vi "ReadStrains_v190627_A.vi"() -> ()   [LabVIEW 2017]
doc: "I. Description:\nThis example demonstrates how to make continuous, hardware-timed temperature measurement using a thermocouple.\n\nII. Instructions for Running:\n1. Specify the Physical Channel where you have connected the thermocouple.\n2. Enter the Minimum and Maximum temperature values in degrees C you expect to measure. A smaller range will allow a more accurate measurement.\n3. Enter the scan rate at which you want to run the acquisition.\n4. Specify the type of thermocouple you are using.\n5. Thermocouple measurements require cold-junction compensation (CJC) to correctly scale them. Specify the source of your cold-junction compensation.\n6. If your CJC source is \"Internal\", skip the rest of the steps.\n7. If your CJC source is \"Constant Value\", specify the value (usually room temperature) in degrees C.\n8. If your CJC source is \"Channel\", specify the CJC Channel name. \n9. Specify the appropriate Auto Zero Mode. See your device's hardware manual to find out if your device supports this attribute.\n\nIII. Block Diagram Steps:\n1. Create a Thermocouple (TC) temperature measurement channel.\n2. Get all the channels in the task.\n3. Convert channel(s) array to a comma-delimited channel string.\n4. This attribute is set to compensate for input offset errors. May not be supported by all devices*.\n5. Call the Timing VI to specify the hardware timing parameters. Use device's internal clock, continuous mode acquisition and the sample rate specified by the user.\n6. Call the Start VI to program and start the acquisition.\n7. Read N samples and plot it. By default, the Read VI reads all available samples, but you can specify how many samples to read at a time and the timeout value. Continue reading data until the stop button is pressed or an error occurs. \n8. Call the Clear Task VI to clear the Task.\n9. Use the popup dialog box to display an error if any.\n\n* If your device does not support Auto Zero Mode bypass Step 2, 3, and 4.\n\nIV. I/O Connections Overview:\nConnect your thermocouple to the terminals corresponding to the Physical Channel I/O Control value."
uses:
  <vilib>/Utility/error.llb/DialogType.ctl
  <vilib>/DAQmx/read.llb/DAQmx Read (Counter DBL 1Chan 1Samp).vi
  <vilib>/DAQmx/write.llb/DAQmx Write (Digital 1D Bool NChan 1Samp 1Line).vi
  <vilib>/DAQmx/read.llb/DAQmx Read (Analog 1D Wfm NChan NSamp).vi
  <vilib>/Analysis/baseanly.llb/Mean (DBL).vi
  <vilib>/DAQmx/create/channels.llb/DAQmx Create Channel (DO-Digital Output).vi
  <vilib>/Waveform/WDTOps.llb/WDT Index Channel DBL.vi
  <vilib>/DAQmx/create/channels.llb/DAQmx Create Channel (AI-Voltage-Basic).vi
  <vilib>/DAQmx/configure/timing.llb/DAQmx Timing (Sample Clock).vi
  <vilib>/DAQmx/create/channels.llb/DAQmx Create Channel (CI-Frequency).vi
  <vilib>/DAQmx/miscellaneous.llb/DAQmx Fill In Error Info.vi
  <vilib>/express/express arith-compare/Formula/XNode/ExpressFormulaBlockNode.xnode
  <vilib>/Analysis/NI_AALBase.lvlib
  <vilib>/ptbypt/NI_PtbyPt.lvlib
  <vilib>/Utility/miscctls.llb/LVRowAndColumnTypeDef.ctl
  <resource>/objmgr/daqmx.rc
panel:
  out "abs(x)":dbl
  in  "Min Frequency":dbl=0.1 format="%0.6f"
  in  "Max Frequency":dbl=50000.0 format="%0.6f"
  in  "Frequency Input Terminal":tag="/Dev1/PFI1"
  out "Freq (Hz)":dbl=5258.660356274239
  in  "Stop":bool
  in  "Counter":tag="Dev1/ctr0"
  in  "Color Box":u32(colorbox)=16448250
  out "Micro-strain":dbl[](array[numeric]) format="%.2g"
  out "Results":i32[](listbox)
  in  "num_chans":i32=4
  in  "Search Strings":string[](array[string])=["Verbose Name", "Units", "Sensitivity", "Offset"]
  out "TRQ_2SPD_OT (N·m)":dbl=-0.01305389404296875 format="%0.3f"
  out "Power_OT (W)":dbl=-4.779110606064606 format="%.2f"
  out "rpm_out/rpm_in":dbl=-8.382425226893735e-05 format="%.3g"
  out "switch_counts":dbl=4500000.0
  in  "switch_time (s)":dbl=900000.0
  out "AI Consumer Iterations":i32=46
  in  "LV_CMD_2SPD_OIL_SLND":bool[](array[boolean])=[FALSE]
  in  "lines":tag="Dev1/port1/line0"
  out "RPM_2SPD_OT_6602":dbl format="%0.1f"
  in  "path":path=path "D:/LabView Data"
  in  "DRVLN_PULLEY_RATIO":dbl=1.48 format="%.2f"
  out "P2 - P1":dbl=2.2560862731933593 format="%.3f"
  out "Recorded Blocks":dbl=46.0
  out "AI Producer Iterations":i32=45
  in  "Force Record":bool caption="Force Record Enable"
  out "RPM_DRVLN_6602":dbl format="%0.1f"
  out "data 2":waveform(dbl)[](array[waveform])=[{"t0"=timestamp(3650018127.9917235 s since 1904-01-01), "dt"=0.1, "Y"=[0.021594634133905076, 0.022275858634939055], "attributes"=variant("NI_ChannelName"=variant(string "Dev1/ai0"), "NI_UnitDescription"=variant(string "Volts"))}, {"t0"=timestamp(3650018127.9917235 s since 1904-01-01), "dt"=0.1, "Y"=[2.0002340930725198, 1.9998772609501023], "attributes"=variant("NI_ChannelName"=variant(string "Dev1/ai0"), "NI_UnitDescription"=variant(string "Volts"))}, {"t0"=timestamp(3650018127.9917235 s since 1904-01-01), "dt"=0.1, "Y"=[1.9878001157523826, 1.9871643057998443], "attributes"=variant("NI_ChannelName"=variant(string "Dev1/ai0"), "NI_UnitDescription"=variant(string "Volts"))}, {"t0"=timestamp(3650018127.9917235 s since 1904-01-01), "dt"=0.1, "Y"=[0.006912624203864532, 0.006889916720453561], "attributes"=variant("NI_ChannelName"=variant(string "Dev1/ai0"), "NI_UnitDescription"=variant(string "Volts"))}, {"t0"=timestamp(3650018127.9917235 s since 1904-01-01), "dt"=0.1, "Y"=[0.0, 0.0], "attributes"=variant("NI_ChannelName"=variant(string "Dev1/ai0"), "NI_UnitDescription"=variant(string "Volts"))}]
  out "Power_IN (W)":dbl=0.0005711775684961294 format="%.2g"
  out "TRQ_2SPD_DRVLN_OT (N·m)":dbl=-0.018612060546874976 format="%0.3f"
  out "Waveform Chart":waveform(dbl)[](graph)=[{"t0"=timestamp(3663084502.027375 s since 1904-01-01), "dt"=0.1, "Y"=[-0.17066702696318498, -0.13693019437081472], "attributes"=variant("NI_ChannelName"=variant(string "HS_2210_STRAIN_A_POUNDS"), "NI_UnitDescription"=variant(string "lbf"))}, {"t0"=timestamp(3663084502.027375 s since 1904-01-01), "dt"=0.1, "Y"=[-50.01120067249004, -50.01071408355846], "attributes"=variant("NI_ChannelName"=variant(string "T1_OIL_OT"), "NI_UnitDescription"=variant(string "°C"))}, {"t0"=timestamp(3663084502.027375 s since 1904-01-01), "dt"=0.1, "Y"=[-0.013838771793185324, -0.013803088604682188], "attributes"=variant("NI_ChannelName"=variant(string "HS_2210_STRAIN_B_VOLTS"), "NI_UnitDescription"=variant(string "V"))}, {"t0"=timestamp(3663084502.027375 s since 1904-01-01), "dt"=0.1, "Y"=[10.033860995992347, 10.033912900500356], "attributes"=variant("NI_ChannelName"=variant(string "HS_2210_EXC_B_VOLTS"), "NI_UnitDescription"=variant(string "V"))}, {"t0"=timestamp(3663084502.027375 s since 1904-01-01), "dt"=0.1, "Y"=[1.48, 1.48], "attributes"=variant("NI_ChannelName"=variant(string "RPM_RATIO"), "NI_UnitDescription"=variant(string "ratio"))}, {"t0"=timestamp(3663084502.027375 s since 1904-01-01), "dt"=0.1, "Y"=[99.0, 99.0], "attributes"=variant("NI_ChannelName"=variant(string "DataTag"), "NI_UnitDescription"=variant(string "none"))}, {"t0"=timestamp(3663084502.027375 s since 1904-01-01), "dt"=0.1, "Y"=[0.0, 0.0], "attributes"=variant("NI_ChannelName"=variant(string "LV_CMD_2SPD_OIL_SLND"), "NI_UnitDescription"=variant(string "boolean"))}]
  in  "Run Letter":string="a"
  out "Recording":bool
  in  "Num_Blocks":dbl=100.0
  in  "Data Tag":dbl=99.0 format="%.2p"
  in  "Maximum Value":dbl=10.0 format="%0.2f"
  in  "Minimum Value":dbl=-10.0 format="%0.2f"
  in  "Physical Channel":tag="Dev1/ai0:3" caption="PCI-6143_1 Channels"
  in  "Rate":dbl=1000.0 format="%0.2f"
  # "rev 150415_A  added \"Record Run X\" sub VI.\nrev 150423_A added power, efficiency, and manual inputs for speed .\nrev 150423_B added speed measurement via PCI-6602 card.\nrev 161117_A is set up for the alternator test reading shaft RPM from Dynapar encoder and torque from the Omega TQ513-1K paired with the Omega DP41-S.\nrev 170504_A migrated DAQ h/w from the SCXI chassis (now being used for TC2 porcupine testing) to PCI-6143.\nrev 170510_A takes data at 1000Hz, then averages groups of 100 samples for a logging rate of 10Hz per channel.  Added function that resets \"Data Tag\"\nto 99 after \"Num_Blocks\" has been recorded.\nrev 170810_A adds flowmeter for 2-speed supercharger drive bench test.  CJP\nrev 170821_A logs tags to same file for a given run letter.  Uses \"Record Continuous Tags...\" sub VI.\nrev 171129_A is for the Orthrus 2-speed drive.  Added new encoder period measurement for the 127 tooth geat \"RPM_2SPD_OT\". CJP\nrev 171130_A adds Digital Output (DO) for 2SPD drive control.  Will log this with the rest of the data.  Also corrected the number of teeth on the 2SPD Output side from 127 to 107!\nrev 171201_A restructuring for  \"real-time\" response to speed changes by moving the disklog to a separate loop (queue).\nrev 171201_B moves counters into main AI loop and adds a start trigger so DAQ won't start until rig is spinning.  Added F-V where old \"F1\" channel was for \"RPM_2SPD_OT\".   CJP\nrev 171201_C uses a CI-Frequency task for RPM instead of period.  Testing this for better transient response.  This appears to be even slower than the period measurement.\nrev 171201_D is built from rev 171201_A, but adding in the F-V channel.  This version queues both the AI channel and CI channels to a single Consumer.  Also adding a 30s switch to automate switching of the 2SPD solenoid.\nrev 171221_A was the first attempt at this and for some reason, while running that VI, the computer froze, unable to do ctrl+alt+del reboot.  After rebooting, the VI was no longer openable in LabView 2014 or LabView 2016.  Will try the same process over with v171226_A.\nrev 171226_A adds one more PCI_6143 card for 8 additional analog inputs.\nrev 171226_B created a backup with 171226_A.\nrev 180314_A added thermocouple for Sumanth.  This is for testing the 2-Speed Drive.\nrev Read \"ThermVolt_TestSpeed_180406_A.vi\" is for verifying the one remaining Micro-Epsilon speed sensor on the 2Spd Drive.\nrev \"Read Thermocouples and Voltages v180406_A.vi\" reintroduces the two counter/timer channels on the PCI-6602 card for the driveline encoder and \nMicro-Epsilon 2Spd Output.\nrev 180919_A built off of rev 180426_A for 2-Speed Drive testing.  CJP\nv181002_A adding new T22 at 2SPD input pulley AND keeping original T22 at output end of drivline.  CJP\nv181004_A corrected front panel displays for Power_IN and Power_OT.  CJP\nv181025_A adding ReadChnCfg.VI to read channel names, units, scaling, and offset from Labview Channel Map\nv190401_A restructuring \"Read Thermocouples and Voltages...\" to use only channels from NI-6229 out of test cell 2.  CJP\nv190516_A adds frequency measurement for driveline speed since F-V measurements not working.  CJP"
  # "For instructions, select Help>>Show Context Help"
  # "Now using 360 PPR encoder for input speed 171227.\nChanged to Input Gear Speed 180118.  CJP  127 Hz = 1 RPS, 127 Hz = 60 RPM\n5 kHz = 1 V => 5000/127 = 39.37 RPS = 2362.205 RPM\nv180314_A 5kHz = 1V = 5000/360 = 13.888 RPS = 833.33 RPM.\nBack to 360PPR encoder with pulley ratio of 1.48."
  # "HBM T21WN"
  # "Interface T22"
  # "Timing Parameters"
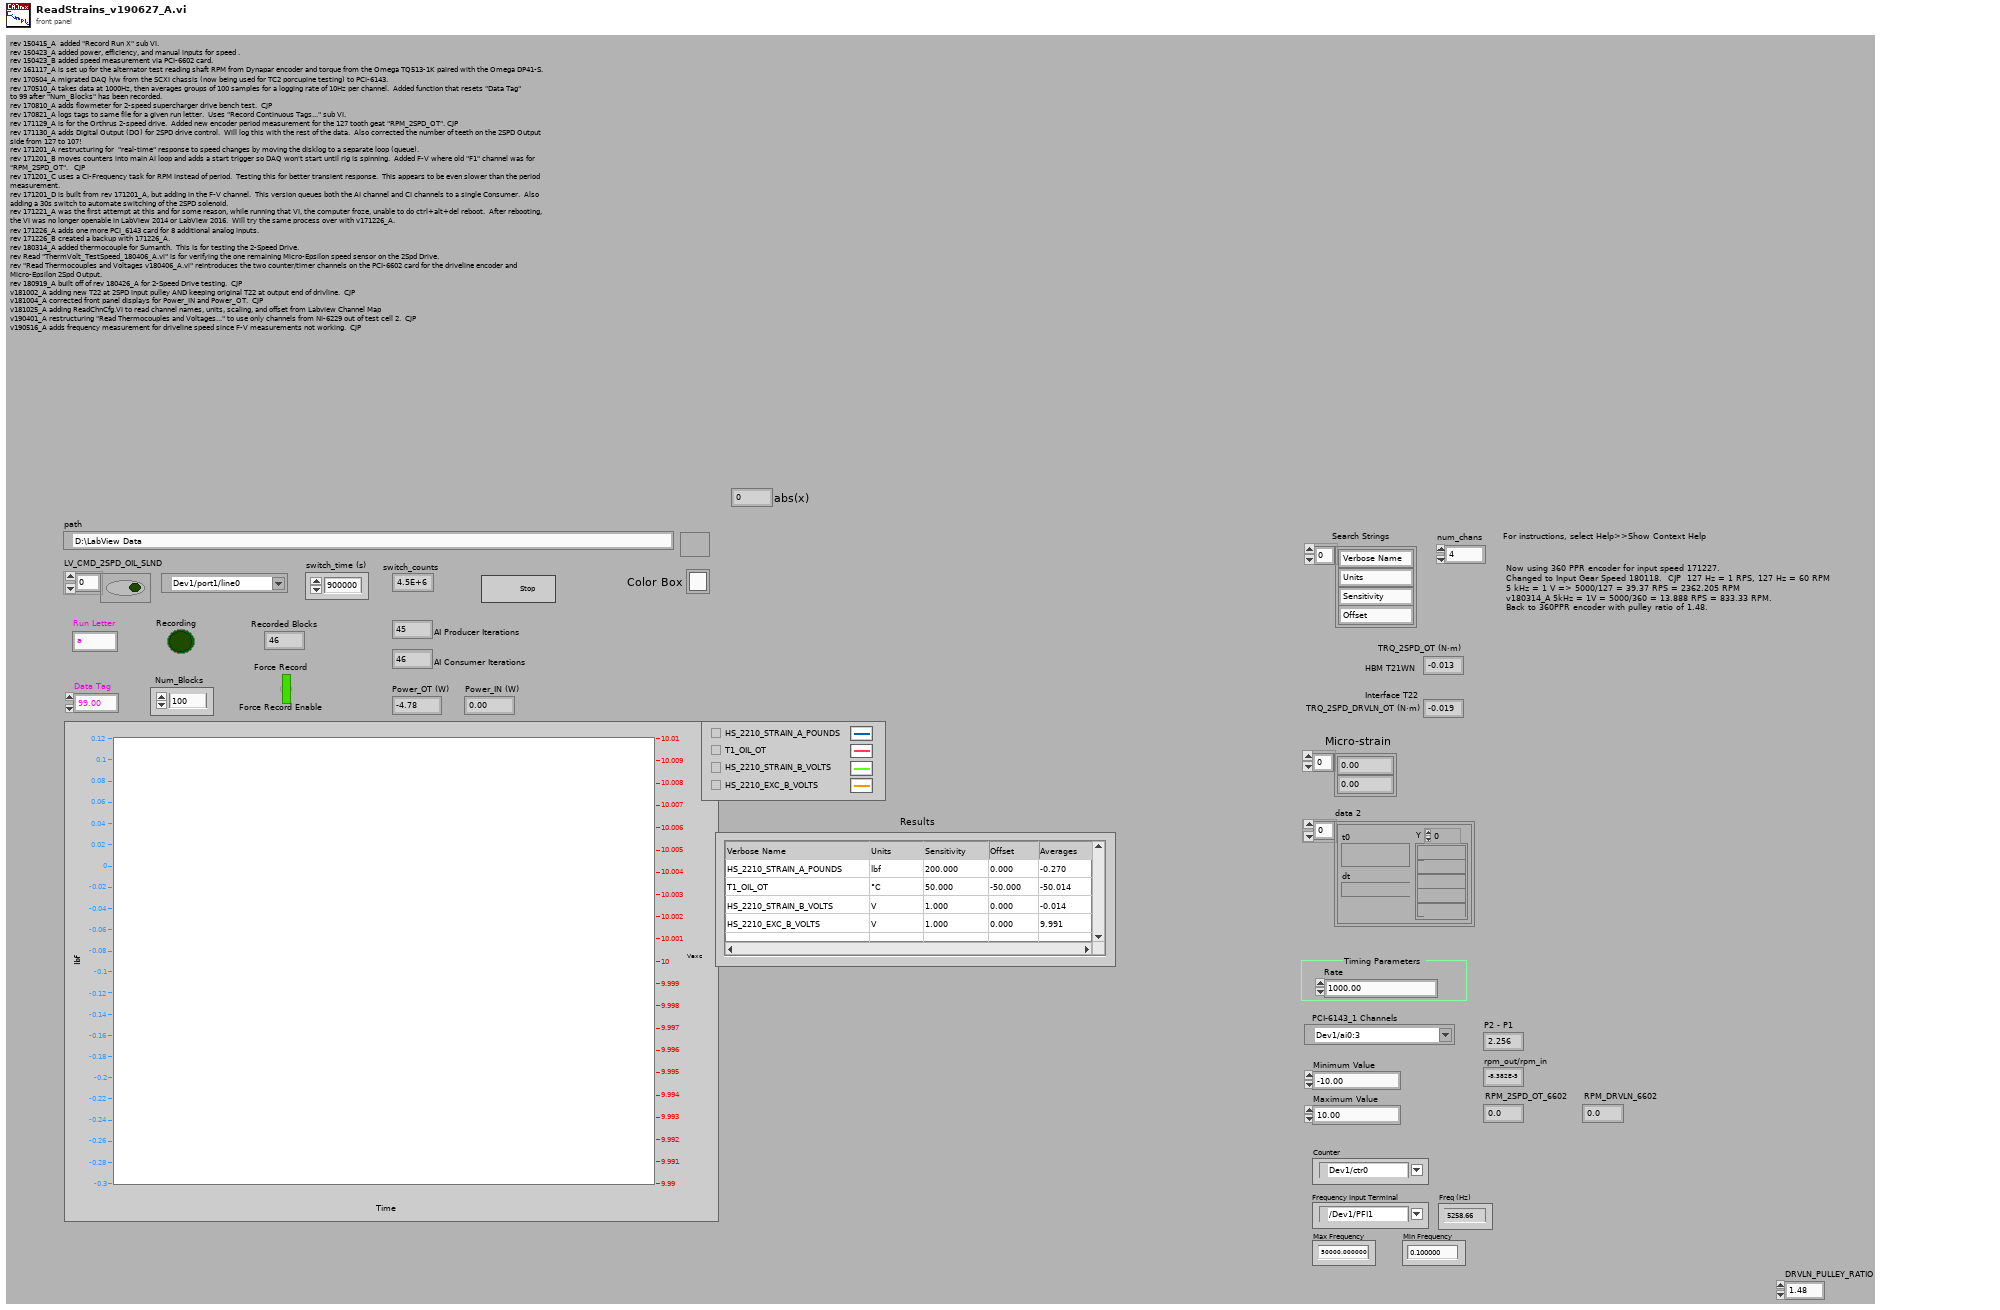
[diagram p1: front panel]
types:
  T1 = typedef "DialogType.ctl" = u16
  T2 = typedef "LVRowAndColumnTypeDef.ctl" = cluster{"Row":i32, "Column":i32}
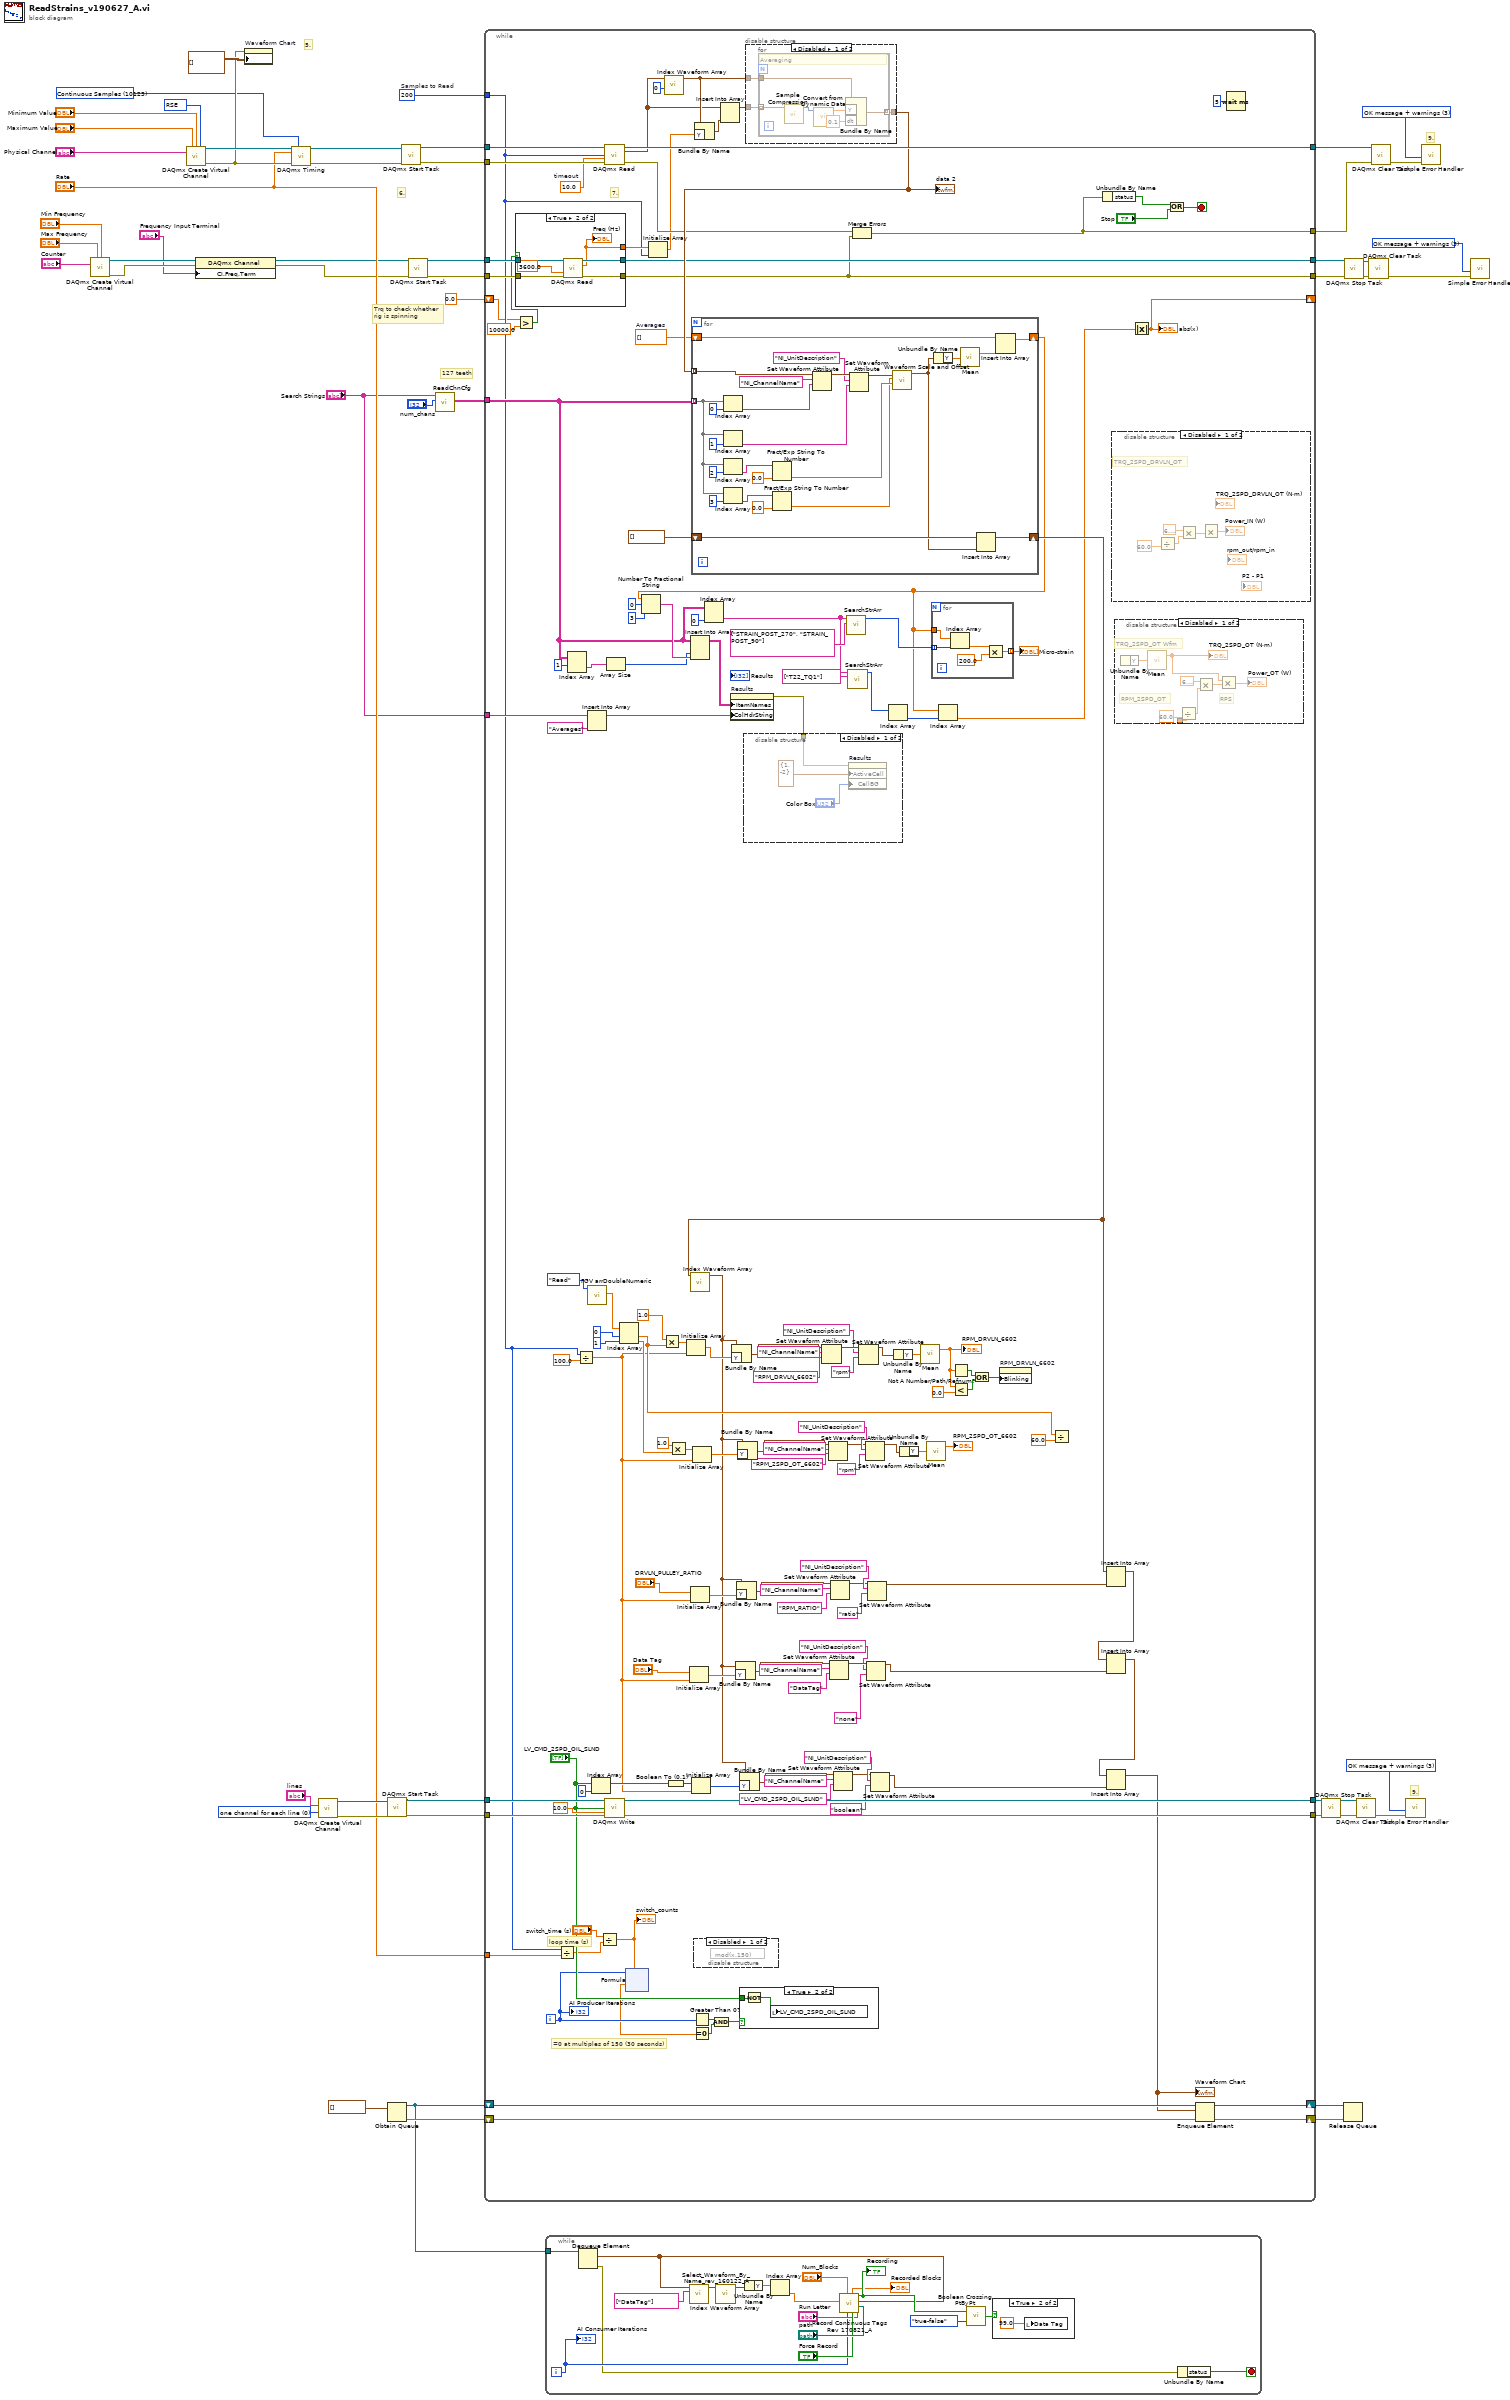
[diagram p0: block diagram]
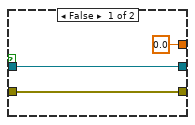
[diagram p4: hidden frame]
diagram:
  w11 = T1 3 items=["no dialog", "OK message", "continue or stop message", "OK message + warnings", "continue/stop + warnings"] ("type of dialog (OK msg:1)")
  w18 = 10083 items=["Default"=-1, "RSE"=10083, "NRSE"=10078, "Differential"=10106, "Pseudodifferential"=12529] ("input terminal configuration")
  w38 = T1 3 items=["no dialog", "OK message", "continue or stop message", "OK message + warnings", "continue/stop + warnings"] ("type of dialog (OK msg:1)")
  w44 = 0 items=["one channel for each line", "one channel for all lines"] ("line grouping")
  w50 = T1 3 items=["no dialog", "OK message", "continue or stop message", "OK message + warnings", "continue/stop + warnings"] ("type of dialog (OK msg:1)")
  w24 = 10123 items=["Finite Samples"=10178, "Continuous Samples"=10123] ("sample mode")
  # "Trq to check whether\nrig is spinning"
  # "127 teeth"
  # "Samples to Read"
  # "9."
  # "9."
  # "5."
  # "6."
  n1 = call-poly <vilib>:"DAQmx Create Virtual Channel.vi"("maximum value"="Max Frequency", "minimum value"="Min Frequency", "counter"="Counter") -> ("task out"=w10:refnum<k21>, "error out"=w9:errorcluster)  [unwired: 11 in]
  n2 = call-poly <vilib>:"DAQmx Create Virtual Channel.vi"("maximum value"="Maximum Value", "minimum value"="Minimum Value", "input terminal configuration"=w18, "physical channels"="Physical Channel") -> ("task out"=w48:refnum<k21>, "error out"=w46:errorcluster)  [unwired: 10 in]
  n3 = property class="DAQmx Channel"(reference=w10, error in=w9, "CI.Freq.Term"="Frequency Input Terminal") -> (reference out=w15:refnum<k21>, error out=w16:errorcluster)
  n4 = property on="Waveform Chart" class="WFChart (strict)"(error in=w46, "History Data"=waveform(dbl)[][] []) -> ()  [unwired: 1 in, 2 out]
  n5 = call-poly <vilib>:"DAQmx Timing.vi"("task/channels in"=w48, "sample mode"=w24, "rate"="Rate", "error in"=w46) -> ("task out"=w51:refnum<k21>, "error out"=w19:errorcluster)  [unwired: 10 in]
  n6 = call-poly <vilib>:"DAQmx Create Virtual Channel.vi"("lines"="lines", "line grouping"=w44) -> ("task out"=w43:refnum<k21>, "error out"=w42:errorcluster)  [unwired: 12 in]
  n7 = call <vilib>:"DAQmx Start Task.vi"("task/channels in"=w43, "error in"=w42) -> ("task out"=w41:refnum<k21>, "error out"=w40:errorcluster)  [unwired: 12 in]
  n8 = Obtain Queue(element data type=waveform(dbl)[] [] ("appended array")) -> (queue out=w28:refnum<queue>, error out=w31:errorcluster)  [unwired: 4 in, 1 out]
  n9 = call <vilib>:"DAQmx Start Task.vi"("task/channels in"=w51, "error in"=w19) -> ("task out"=w53:refnum<k21>, "error out"=w54:errorcluster)  [unwired: 12 in]
  n10 = call <vilib>:"DAQmx Start Task.vi"("task/channels in"=w15, "error in"=w16) -> ("task out"=w5:refnum<k21>, "error out"=w4:errorcluster)  [unwired: 12 in]
  n11 = call "ReadChnCfg.vi"("num_chans"="num_chans", "Search Strings"="Search Strings") -> ("Table Minus Headers"=w22:string[][])  [unwired: 8 in, 1 out]
  n12 = while {
    tunnel: w53 -> [w196]
    tunnel: w54 -> [w195]
    tunnel: [w194] -> w52
    tunnel: 200 ("number of samples per channel") -> [w71]
    tunnel: w41 -> [w142]
    tunnel: w40 -> [w141]
    tunnel: [w140] -> w35
    tunnel: [w139] -> w34
    shift-right: [w125] -> w30
    shift-left: w28 -> [w127]
    shift-right: [w124] -> w29
    shift-left: w31 -> [w126]
    tunnel: "Rate" -> [w118]
    tunnel: [w76] -> w20
    tunnel: w22 -> [w85]
    tunnel: "Search Strings" -> [w95]
    tunnel: w5 -> [w79]
    tunnel: w4 -> [w78]
    tunnel: [w75] -> w3
    tunnel: [w74] -> w2
    shift-right: [w59] -> _
    shift-left: 0.0 -> [w58]
    i -> [w115]
    stop <- w191 stop-if-true
    w106 = dbl[] []  # Averages
    w192 = 10.0  # timeout
    # "loop time (s)"
    # "=0 at multiples of 150 (30 seconds)"
    # "7."
    n13 = Greater?(x=w58, y=10000.0) -> (0:w56:bool)
    n14 = case shown="True" w56 {
      tunnel: w79 -> [w209 w215]
      tunnel: w78 -> [w208 w214]
      tunnel: [w209 w213] -> w75
      tunnel: [w208 w212] -> w74
      tunnel: [0.0 ("data") w210] -> w72
      frame False {
      }
      frame True {
        n15 = call-poly <vilib>:"DAQmx Read.vi"("task/channels in"=w215, "timeout"=3600.0, "error in"=w214) -> ("task out"=w213:refnum<k21>, "data"=w210:dbl, "error out"=w212:errorcluster)  [unwired: 10 in]
        "Freq (Hz)" <- w210
      }
    }
    n16 = Divide(x=w71, y=w118) -> (x/y=w117:dbl)
    n17 = Index Array(array=w85, index (row)=1) -> (element=w89:string[])  [unwired: 1 in]
    n18 = Divide(x=w71, y=100.0) -> (x/y=w128:dbl)
    n19 = Insert Into Array(array=w95, new element="Averages" ("new element/subarray")) -> (w86:string[])  [unwired: 1 in]
    n20 = call "FGV arrDoubleNumeric.vi"("Enum"=enum16{"Read", "Write"}."Read") -> ("Array OUT"=w157:dbl[])  [unwired: 9 in, 1 out]
    n21 = Index Array(array="LV_CMD_2SPD_OIL_SLND", index=0) -> (element=w136:bool)
    n22 = Divide(x="switch_time (s)", y=w117) -> (x/y=w114:dbl)
    "switch_counts" <- w114
    n23 = call-poly <vilib>:"DAQmx Read.vi"("task/channels in"=w196, "number of samples per channel"=w71, "timeout"=w192, "error in"=w195) -> ("task out"=w194:refnum<k21>, "data"=w68:waveform(dbl)[], "error out"=w77:errorcluster)  [unwired: 9 in]
    n24 = call-poly <vilib>:"DAQmx Write.vi"("task/channels in"=w142, "data"="LV_CMD_2SPD_OIL_SLND", "timeout"=10.0, "error in"=w141) -> ("task out"=w140:refnum<k21>, "error out"=w139:errorcluster)  [unwired: 9 in, 1 out]
    n25 = Array Size(array=w89) -> (size(s)=w88:i32)
    n26 = Index Array(array=w157, index #1=0 ("index"), index #2=1 ("index")) -> (element #1=w156:dbl, element #2=w143:dbl)
    n27 = xnode "Formula"("X1"=w115, "X2"=w114) -> ("Result"=w113:dbl)  [unwired: 1 in, 1 out]
    n28 = Initialize Array(w72, w71) -> (w70:dbl[])
    n29 = Multiply(x=1.0, y=w156) -> (x*y=w174:dbl)
    n30 = call-poly <vilib>:"Index Waveform Array.vi"("index"=0, "waveform array"=w68) -> ("waveform"=w69:waveform(dbl))  [unwired: 8 in, 1 out]
    n31 = Boolean To (0,1)(Boolean=w136) -> (0, 1=w129:i16)
    n32 = Multiply(x=1.0, y=w143) -> (x*y=w151:dbl)
    n33 = Initialize Array(w174, w128) -> (w181:dbl[])
    n34 = Initialize Array("Data Tag", w128) -> (w159:dbl[])
    n35 = Initialize Array("DRVLN_PULLEY_RATIO", w128) -> (w172:dbl[])
    n36 = Initialize Array(w129, w128) -> (w123:i16[])
    n37 = Initialize Array(w151, w128) -> (w150:dbl[])
    n38 = Greater Than 0?(x=w115) -> (x > 0?=w120:bool)
    n39 = Equal To 0?(x=w113) -> (x = 0?=w119:bool)
    n40 = disable-structure shown="Disabled" {
      frame Disabled {
        n41 = expression code="mod(x,150)"() -> ()  [unwired: 1 in, 1 out]
      }
      frame Enabled {
      }
    }
    n42 = Bundle By Name(cluster=w69, "Y"=w70) -> (w67:waveform(dbl))
    n43 = Index Array(array=w85, index (col)=0 ("disabled index (col)")) -> (element=w65:string[])  [unwired: 1 in]
    n44 = And(x=w120, y=w119) -> (x .and. y?=w121:bool)
    n45 = Insert Into Array(array=w68, new element=w67) -> (w66:waveform(dbl)[])  [unwired: 1 in]
    n46 = case shown="True" w121 {
      tunnel: "LV_CMD_2SPD_OIL_SLND" -> [_ w273]
      frame False {
      }
      frame True {
        n47 = Not(x=w273) -> (.not. x?=w272:bool[])
        n48 = local write "LV_CMD_2SPD_OIL_SLND"(w272) -> ()
      }
    }
    n49 = disable-structure shown="Disabled" {
      disable-tunnel: [w199 w206] -> w108
      disable-tunnel: w69 -> [w198 _]
      disable-tunnel: w66 -> [w197 w206]
      frame Disabled {
        n50 = for {
          tunnel: w197 -> [w202] mode=indexing
          tunnel: [w201] -> w199 mode=indexing
          tunnel: w198 -> [w200]
          # "Averaging"
          n51 = call "Sample Compression"("Signals"=w202) -> ("Mean"=w203:dynamicdata)  [unwired: 8 in, 2 out]
          n52 = call "Convert from Dynamic Data"("Dynamic Data Type"=w203) -> ("Array"=w205:dbl[])  [unwired: 3 in]
          n53 = Bundle By Name(cluster=w200, "Y"=w205, "dt"=0.1) -> (w201:waveform(dbl))
        }
      }
      frame Enabled {
      }
    }
    "data 2" <- w108
    n54 = for {
      tunnel: w108 -> [w248] mode=indexing
      shift-right: [w247] -> w63
      shift-left: w106 -> [w246]
      tunnel: w85 -> [w235] mode=indexing
      shift-right: [w242] -> w102
      shift-left: waveform(dbl)[] [] -> [w244]
      n55 = Index Array(array=w235, index=0) -> (element=w239:string)
      n56 = Index Array(array=w235, index=1) -> (element=w238:string)
      n57 = Index Array(array=w235, index=2) -> (element=w234:string)
      n58 = Index Array(array=w235, index=3) -> (element=w230:string)
      n59 = Fract/Exp String To Number(string=w234, default (0 dbl)=0.0) -> (number=w232:dbl)  [unwired: 2 in, 1 out]
      n60 = Fract/Exp String To Number(string=w230, default (0 dbl)=0.0) -> (number=w229:dbl)  [unwired: 2 in, 1 out]
      n61 = Set Waveform Attribute(5:w239, 6:"NI_ChannelName" ("name"), 7:w248) -> (3:w252:waveform(dbl))  [unwired: 1 in, 2 out]
      n62 = Set Waveform Attribute(5:w238, 6:"NI_UnitDescription" ("name"), 7:w252) -> (3:w250:waveform(dbl))  [unwired: 1 in, 2 out]
      n63 = call <vilib>:"Waveform Scale and Offset.vi"("scale"=w232, "offset"=w229, "waveform in"=w250) -> ("waveform out"=w243:waveform(dbl))  [unwired: 7 in, 1 out]
      n64 = Unbundle By Name(w243) -> ("Y"=w249:dbl[])
      n65 = call-poly <vilib>:"Mean.vi"("X"=w249) -> ("mean"=w245:dbl)  [unwired: 1 out]
      n66 = Insert Into Array(array=w244, new element=w243) -> (w242:waveform(dbl)[])  [unwired: 1 in]
      n67 = Insert Into Array(array=w246, new element=w245) -> (w247:dbl[])  [unwired: 1 in]
    }
    n68 = Number To Fractional String(number=w63, width (-)=i16 0, precision (6)=i16 3) -> (F-format string=w91:string[])  [unwired: 1 in]
    n69 = Insert Into Array(array=w85, index (col)=w88, new element=w91) -> (w87:string[][])  [unwired: 1 in]
    n70 = call-poly <vilib>:"Index Waveform Array.vi"("waveform array"=w102) -> ("waveform"=w103:waveform(dbl))  [unwired: 9 in, 1 out]
    n71 = property on="Results" class="MCListbox (strict)"("ItemNames"=w87, "ColHdrString"=w86) -> (error out=w80:errorcluster)  [unwired: 2 in, 1 out]
    n72 = Bundle By Name(cluster=w103, "Y"=w181) -> (w173:waveform(dbl))
    n73 = Bundle By Name(cluster=w103, "Y"=w159) -> (w165:waveform(dbl))
    n74 = Bundle By Name(cluster=w103, "Y"=w172) -> (w166:waveform(dbl))
    n75 = Bundle By Name(cluster=w103, "Y"=w150) -> (w152:waveform(dbl))
    n76 = Bundle By Name(cluster=w103, "Y"=w123) -> (w130:waveform(dbl))
    n77 = disable-structure shown="Disabled" {
      disable-tunnel: w80 -> [w218 _]
      frame Disabled {
        n78 = property on="Results" class="MCListbox (strict)"(error in=w218, "ActiveCell"=T2 {"Row"=1, "Column"=-2} ("Active Cell:Active Cell"), "CellBG"="Color Box") -> ()  [unwired: 1 in, 2 out]
      }
      frame Enabled {
      }
    }
    n79 = Set Waveform Attribute(5:"RPM_DRVLN_6602" ("name"), 6:"NI_ChannelName" ("name"), 7:w173) -> (3:w185:waveform(dbl))  [unwired: 1 in, 2 out]
    n80 = Set Waveform Attribute(5:"RPM_2SPD_OT_6602" ("name"), 6:"NI_ChannelName" ("name"), 7:w152) -> (3:w146:waveform(dbl))  [unwired: 1 in, 2 out]
    n81 = Set Waveform Attribute(5:"DataTag" ("name"), 6:"NI_ChannelName" ("name"), 7:w165) -> (3:w163:waveform(dbl))  [unwired: 1 in, 2 out]
    n82 = Set Waveform Attribute(5:"RPM_RATIO" ("name"), 6:"NI_ChannelName" ("name"), 7:w166) -> (3:w168:waveform(dbl))  [unwired: 1 in, 2 out]
    n83 = Set Waveform Attribute(5:"LV_CMD_2SPD_OIL_SLND" ("name"), 6:"NI_ChannelName" ("name"), 7:w130) -> (3:w132:waveform(dbl))  [unwired: 1 in, 2 out]
    n84 = call "SearchStrArr.vi"("asSearchList"=string[] ["STRAIN_POST_270", "STRAIN_POST_90"], "asDict"=w65) -> ("aiRowIdx"=w82:i32[])  [unwired: 9 in]
    n85 = call "SearchStrArr.vi"("asSearchList"=string[] ["T22_TQ1"], "asDict"=w65) -> ("aiRowIdx"=w62:i32[])  [unwired: 9 in]
    n86 = Merge Errors(w77, w74) -> (w76:errorcluster)
    n87 = Set Waveform Attribute(5:"rpm" ("name"), 6:"NI_UnitDescription" ("name"), 7:w185) -> (3:w104:waveform(dbl))  [unwired: 1 in, 2 out]
    n88 = Set Waveform Attribute(5:"rpm" ("name"), 6:"NI_UnitDescription" ("name"), 7:w146) -> (3:w109:waveform(dbl))  [unwired: 1 in, 2 out]
    n89 = Set Waveform Attribute(5:"none" ("name"), 6:"NI_UnitDescription" ("name"), 7:w163) -> (3:w97:waveform(dbl))  [unwired: 1 in, 2 out]
    n90 = Set Waveform Attribute(5:"ratio" ("name"), 6:"NI_UnitDescription" ("name"), 7:w168) -> (3:w101:waveform(dbl))  [unwired: 1 in, 2 out]
    n91 = Set Waveform Attribute(5:"boolean" ("name"), 6:"NI_UnitDescription" ("name"), 7:w132) -> (3:w96:waveform(dbl))  [unwired: 1 in, 2 out]
    n92 = Index Array(array=w62) -> (element=w61:i32)  [unwired: 1 in]
    n93 = Unbundle By Name(w104) -> ("Y"=w182:dbl[])
    n94 = Unbundle By Name(w109) -> ("Y"=w149:dbl[])
    n95 = call-poly <vilib>:"Mean.vi"("X"=w182) -> ("mean"=w111:dbl)  [unwired: 1 out]
    "RPM_DRVLN_6602" <- w111
    n96 = call-poly <vilib>:"Mean.vi"("X"=w149) -> ("mean"=→"RPM_2SPD_OT_6602":dbl)  [unwired: 1 out]
    n97 = for {
      tunnel: w82 -> [w222] mode=indexing
      tunnel: w63 -> [w223]
      tunnel: [w219] -> w81 mode=indexing
      n98 = Index Array(array=w223, index=w222) -> (element=w221:dbl)
      n99 = Multiply(x=w221, y=200.0) -> (x*y=w219:dbl)
    }
    "Micro-strain" <- w81
    n100 = Index Array(array=w63, index=w61) -> (element=w60:dbl)
    n101 = Not A Number/Path/Refnum?(number/path/refnum=w111) -> (NaN/Path/Refnum?=w179:bool)
    n102 = Less?(x=w111, y=0.0) -> (x < y?=w180:bool)
    n103 = Or(x=w179, y=w180) -> (x .or. y?=w177:bool)
    n104 = property on="RPM_DRVLN_6602" class="DigNum (strict)"("Blinking"=w177) -> ()  [unwired: 2 in, 2 out]
    n105 = Divide(x=w156, y=60.0) -> ()  [unwired: 1 out]
    n106 = Unbundle By Name(w76) -> ("status"=w193:bool)
    n107 = Insert Into Array(array=w102, new element=w101) -> (w100:waveform(dbl)[])  [unwired: 1 in]
    n108 = Insert Into Array(array=w100, new element=w97) -> (w99:waveform(dbl)[])  [unwired: 1 in]
    n109 = Insert Into Array(array=w99, new element=w96) -> (w98:waveform(dbl)[])  [unwired: 1 in]
    "Waveform Chart" <- w98
    n110 = disable-structure shown="Disabled" {
      frame Disabled {
        # "TRQ_2SPD_DRVLN_OT"
        n111 = Divide(y=60.0) -> (x/y=w224:dbl)  [unwired: 1 in]
        n112 = Multiply(x=6.283185307179586, y=w224) -> (x*y=w227:dbl)
        n113 = Multiply(y=w227) -> (x*y=→"Power_IN (W)":dbl)  [unwired: 1 in]
      }
      frame Enabled {
      }
    }
    n114 = disable-structure shown="Disabled" {
      disable-tunnel: _ -> [w254 _]
      frame Disabled {
        # "RPM_2SPD_OT"
        # "TRQ_2SPD_OT Wfm"
        # "RPS"
        n115 = Unbundle By Name() -> ("Y"=w258:dbl[])  [unwired: 1 in]
        n116 = call-poly <vilib>:"Mean.vi"("X"=w258) -> ("mean"=w257:dbl)  [unwired: 1 out]
        "TRQ_2SPD_OT (N·m)" <- w257
        n117 = Divide(x=w254, y=60.0) -> (x/y=w255:dbl)
        n118 = Multiply(x=6.283185307179586, y=w255) -> (x*y=w260:dbl)
        n119 = Multiply(x=w257, y=w260) -> (x*y=→"Power_OT (W)":dbl)
      }
      frame Enabled {
      }
    }
    n120 = Absolute Value(x=w60) -> (abs(x)=w59:dbl)
    "abs(x)" <- w59
    n121 = Or(x=w193, y="Stop") -> (x .or. y?=w191:bool)
    n122 = Enqueue Element(queue=w127, element=w98, error in (no error)=w126) -> (queue out=w125:refnum<queue>, error out=w124:errorcluster)  [unwired: 1 in, 1 out]
    n123 = Wait (ms)(milliseconds to wait=u32 5) -> ()  [unwired: 1 out]
    "AI Producer Iterations" <- w115
  }
  n124 = while {
    tunnel: w28 -> [w283]
    i -> [w282]
    stop <- w274 stop-if-true
    n125 = Dequeue Element(queue=w283) -> (element=w277:waveform(dbl)[], error out=w275:errorcluster)  [unwired: 2 in, 2 out]
    n126 = call "Select_Waveform_By_Name_rev_160122_A.vi"("Array"=string[] ["DataTag"], "Waveform Array"=w277) -> ("Array 2"=w280:waveform(dbl)[])  [unwired: 9 in]
    n127 = call-poly <vilib>:"Index Waveform Array.vi"("waveform array"=w280) -> ("waveform"=w279:waveform(dbl))  [unwired: 9 in, 1 out]
    n128 = Unbundle By Name(w279) -> ("Y"=w278:dbl[])
    n129 = Index Array(array=w278) -> (element=w276:dbl)  [unwired: 1 in]
    n130 = call "Record Continuous Tags Rev 170821_A.vi"("Run Letter"="Run Letter", "path"="path", "Waveform Array In"=w277, "Force Record"="Force Record", "Main Count"=w282, "Num_Blocks"="Num_Blocks", "Data Tag"=w276) -> ("Record Cmd"=w289:bool, "Recorded Blocks"=→"Recorded Blocks":dbl)  [unwired: 2 in, 1 out]
    "Recording" <- w289
    n131 = call <vilib>:"Boolean Crossing PtByPt.vi"("direction"=enum16{"either", "false-true", "true-false"}."true-false", "input"=w289) -> ("crossing"=w290:bool)  [unwired: 1 in]
    n132 = case shown="True" w290 {
      frame False {
      }
      frame True {
        n133 = local write "Data Tag"(99.0 ("y")) -> ()
      }
    }
    n134 = Unbundle By Name(w275) -> ("status"=w274:bool)
    "AI Consumer Iterations" <- w282
  }
  n135 = call <vilib>:"DAQmx Stop Task.vi"("task/channels in"=w35, "error in"=w34) -> ("task out"=w37:refnum<k21>, "error out"=w36:errorcluster)  [unwired: 12 in]
  n136 = Release Queue(queue=w30, error in (no error)=w29) -> ()  [unwired: 1 in, 3 out]
  n137 = call <vilib>:"DAQmx Stop Task.vi"("task/channels in"=w3, "error in"=w2) -> ("task out"=w13:refnum<k21>, "error out"=w12:errorcluster)  [unwired: 12 in]
  n138 = call <vilib>:"DAQmx Clear Task.vi"("task in"=w37, "error in"=w36) -> ("error out"=w39:errorcluster)  [unwired: 13 in]
  n139 = call <vilib>:"DAQmx Clear Task.vi"("task in"=w13, "error in"=w12) -> ("error out"=w14:errorcluster)  [unwired: 13 in]
  n140 = call <vilib>:"DAQmx Clear Task.vi"("task in"=w52, "error in"=w20) -> ("error out"=w55:errorcluster)  [unwired: 13 in]
  n141 = call <vilib>:"Simple Error Handler.vi"("type of dialog (OK msg:1)"=w38, "error in (no error)"=w39) -> ()  [unwired: 3 in, 5 out]
  n142 = call <vilib>:"Simple Error Handler.vi"("type of dialog (OK msg:1)"=w50, "error in (no error)"=w55) -> ()  [unwired: 3 in, 5 out]
  n143 = call <vilib>:"Simple Error Handler.vi"("type of dialog (OK msg:1)"=w11, "error in (no error)"=w14) -> ()  [unwired: 3 in, 5 out]
